vi "worksheet set start page.vi"(8 "error in (no error)":errorcluster, 10 "start_page":u16, 11 "worksheet":u32) -> (0 "error out":errorcluster)   [LabVIEW 2015, in "xlsxwriter.lvlib"]
doc: "void worksheet_set_start_page(lxw_worksheet worksheet, uint16_t start_page);"
uses:
  xlsxwriter.lvlib
  xlsxwriter.dll
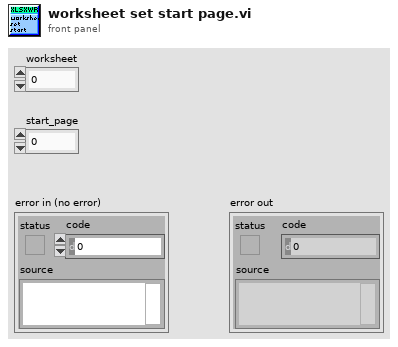
[diagram p1: front panel]
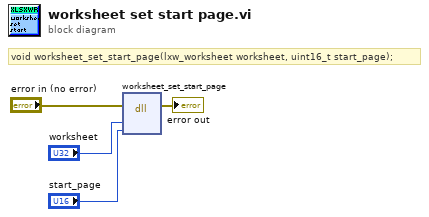
[diagram p0: block diagram]
diagram:
  # "void worksheet_set_start_page(lxw_worksheet worksheet, uint16_t start_page);"
  n1 = dll-call lib="C:/Users/WDAGUtilityAccount/Desktop/lv_vis_added_cell/xlsxwriter.*" fn="worksheet_set_start_page"(error in="error in (no error)", "worksheet"="worksheet", "start_page"="start_page") -> (error out=→"error out":errorcluster)  [unwired: 5 in, 1 out]
